vi "ScaleTraj_LengthAnterior.vi"(8 "Enum":enum16{"3D", "2D"}(ring)=enum."2D", 10 "ScalingCoef":dbl=1.0, 11 "Averaged Gait":dbl[][](array[numeric])) -> (2 "ScaledGait":dbl[][](array[numeric]), 3 "XY Graph":cluster{"Y":dbl[], "Y":dbl[]}[](graph))   [LabVIEW 2016]
uses:
  <userlib>/_OpenG.lib/array/array.llb/Index 1D Array Elements (DBL)__ogtk.vi
  <vilib>/imath/engines/lvmath2/RunTimeEngine/IndexRead/NIMS V(S).vi
  <instcachedir>/0/NIMS V(S)_0488751826AF41519A22953C041130DC.lvgen/NIMS V(S)_0488751826AF41519A22953C041130DC_000.vi
  <vilib>/imathl/engines/lvmath/Functions/Error Handling/Create Error.vi
  <vilib>/imath/engines/lvmath2/RunTimeEngine/ArithmeticOperatorToken/NIMS_ArithmeticOperator_power(S).vi
  <instcachedir>/0/NIMS_ArithmeticOperator_power(S)_1E6AB98FD36540B9B758A69A385A1B47.lvgen/NIMS_ArithmeticOperator_power(S)_1E6AB98FD36540B9B758A69A385A1B47_015.vi
  <instcachedir>/0/NIMS_ArithmeticOperator_power(S)_1E6AB98FD36540B9B758A69A385A1B47.lvgen/NIMS_ArithmeticOperator_power(S)_1E6AB98FD36540B9B758A69A385A1B47_014.vi
  <vilib>/imath/engines/lvmath2/RunTimeEngine/ErrorHandling/NIMS_Create Error From Enums.vi
  <vilib>/imath/engines/lvmath2/RunTimeEngine/NodeEndStatement/NIMS_NodeEndStatement_Output.vi
  <instcachedir>/0/NIMS_NodeEndStatement_Output_53EC0D466D134D7ABD903AC30B43404B.lvgen/NIMS_NodeEndStatement_Output_53EC0D466D134D7ABD903AC30B43404B_005.vi
  <vilib>/imath/engines/lvmath2/RunTimeEngine/ErrorHandling/NIMS_Finalize Error.vi
panel:
  out "XY Graph 2":cluster{dbl[], "yi":dbl[]}(graph)
  out "XY":cluster{"Mean":dbl[], "Mean":dbl[]}[](array[cluster])
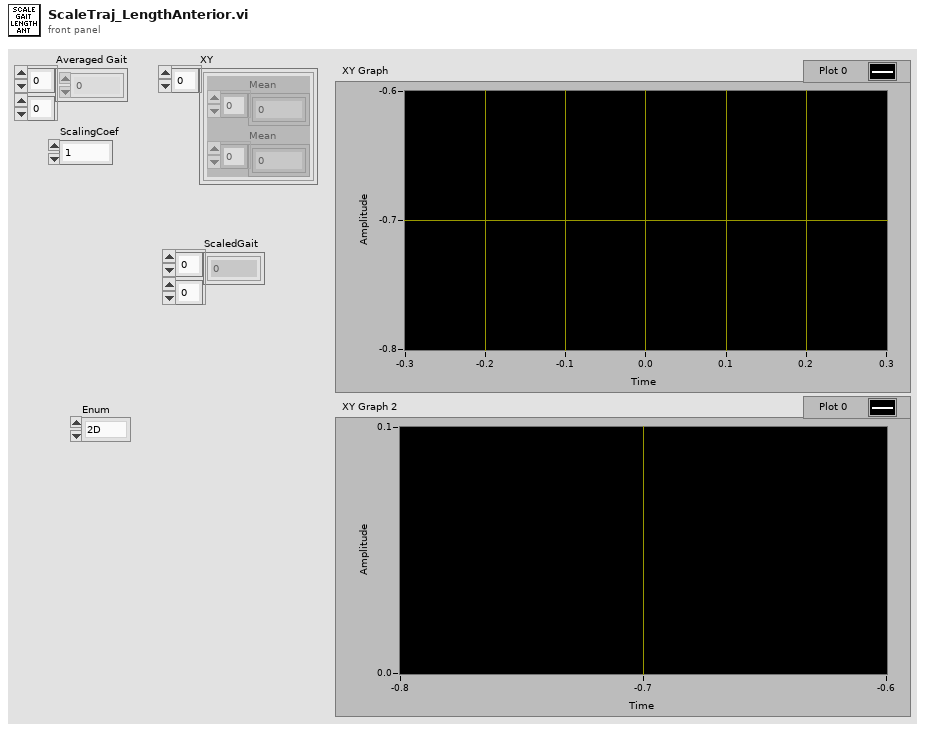
[diagram p1: front panel]
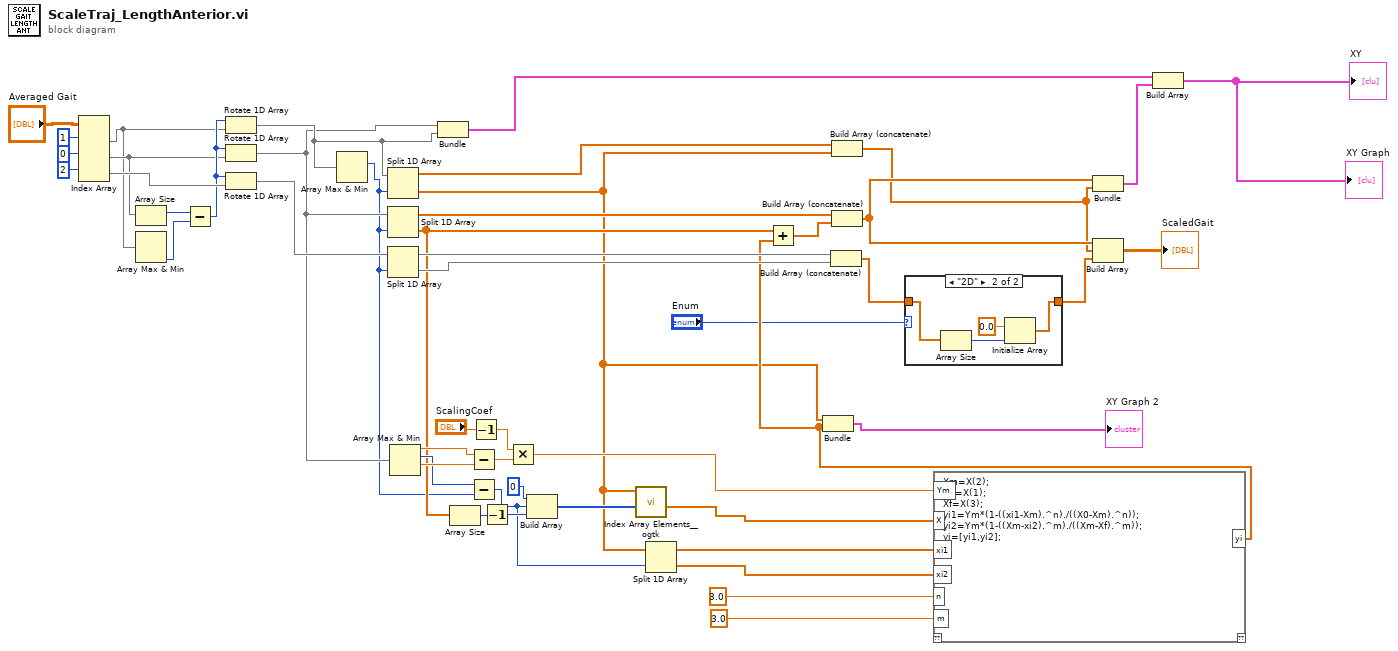
[diagram p0: block diagram]
diagram:
  n1 = Index Array(array="Averaged Gait", index (row) #1=1 ("index (row)"), index (row) #2=0 ("index (row)"), index (row) #3=2 ("index (row)")) -> (element #1=w3:dbl[], element #2=w4:dbl[], element #3=w43:dbl[])  [unwired: 3 in]
  n2 = Array Size(array=w4) -> (size(s)=w45:i32)
  n3 = Array Max & Min(array=w3) -> (min index (indices)=w1:i32)  [unwired: 3 out]
  n4 = Subtract(x=w45, y=w1) -> (x-y=w42:i32)
  n5 = Rotate 1D Array(1:w3, 2:w42) -> (0:w6:dbl[])
  n6 = Rotate 1D Array(1:w4, 2:w42) -> (0:w5:dbl[])
  n7 = Rotate 1D Array(1:w43, 2:w42) -> (0:w40:dbl[])
  n8 = Array Max & Min(array=w6) -> (max index (indices)=w2:i32)  [unwired: 3 out]
  n9 = Split 1D Array(array=w6, index=w2) -> (first subarray=w33:dbl[], second subarray=w17:dbl[])
  n10 = Split 1D Array(array=w5, index=w2) -> (first subarray=w34:dbl[], second subarray=w24:dbl[])
  n11 = Split 1D Array(array=w40, index=w2) -> (first subarray=w32:dbl[], second subarray=w31:dbl[])
  n12 = Array Max & Min(array=w5) -> (max value=w36:dbl, max index (indices)=w28:i32, min value=w37:dbl)  [unwired: 1 out]
  n13 = Bundle(w5, w6) -> (w49:cluster{dbl[], dbl[]})  [unwired: 1 in]
  n14 = Array Size(array=w24) -> (size(s)=w39:i32)
  n15 = Subtract(x=w36, y=w37) -> (x-y=w26:dbl)
  n16 = Subtract(x=w28, y=w2) -> (x-y=w16:i32)
  n17 = Decrement(x="ScalingCoef") -> (x-1=w25:dbl)
  n18 = Decrement(x=w39) -> (x-1=w27:i32)
  n19 = Multiply(x=w25, y=w26) -> (x*y=w21:dbl)
  n20 = Build Array(0 ("element"), w16, w27) -> (w22:i32[])
  n21 = call-poly <userlib>:"Index Array Elements__ogtk.vi"("indices"=w22, "array"=w17) -> ("elements"=w20:dbl[])  [unwired: 9 in]
  n22 = Split 1D Array(array=w17, index=w16) -> (first subarray=w15:dbl[], second subarray=w14:dbl[])
  n23 = Build Array (concatenate)(w32, w31) -> (w10:dbl[])
  n24 = Build Array (concatenate)(w33, w17) -> (w7:dbl[])
  n25 = case shown="\"2D\"" "Enum" {
    tunnel: w10 -> [w50 w54]
    tunnel: [w50 w52] -> w9
    frame "3D", Default {
    }
    frame "2D" {
      n26 = Array Size(array=w54) -> (size(s)=w53:i32)
      n27 = Initialize Array(0.0 ("element"), w53) -> (w52:dbl[])
    }
  }
  n28 = mathscript code="Xm=X(2);\nX0=X(1);\nXf=X(3);\nyi1=Ym*(1-((xi1-Xm).^n)./((X0-Xm).^n));\nyi2=Ym*(1-((Xm-xi2).^m)./((Xm-Xf).^m));\nyi=[yi1,yi2];"("Ym"=w21, "X"=w20, "xi1"=w15, "n"=3.0 ("element"), "xi2"=w14, "m"=3.0 ("element")) -> ("yi"=w18:dbl[])  [unwired: 1 in, 1 out]
  n29 = Add(x=w24, y=w18) -> (x+y=w35:dbl[])
  n30 = Bundle(w17, "yi"=w18) -> (→"XY Graph 2":cluster{dbl[], "yi":dbl[]})  [unwired: 1 in]
  n31 = Build Array (concatenate)(w34, w35) -> (w8:dbl[])
  n32 = Bundle(w8, w7) -> (w30:cluster{dbl[], dbl[]})  [unwired: 1 in]
  n33 = Build Array(w8, w7, w9) -> (→"ScaledGait":dbl[][])
  n34 = Build Array(w49, w30) -> (→"XY" →"XY Graph":cluster{dbl[], dbl[]}[])
